vi "WFM MNGR Initialize ET Waveforms.vi"(8 "error in (no error)":errorcluster, 10 "Sequence File":refnum<k7>, 11 "WFM MNGR in":refnum<class "QPA MSMT Waveform Manager.lvclass">) -> (0 "error out":errorcluster, 3 "WFM MNGR out":refnum<class "QPA MSMT Waveform Manager.lvclass">)   [LabVIEW 2016, in "QPA MSMT Waveform Manager.lvclass"]
uses:
  QPA MSMT Waveform Manager.lvclass
  Controls/ET Waveform.ctl
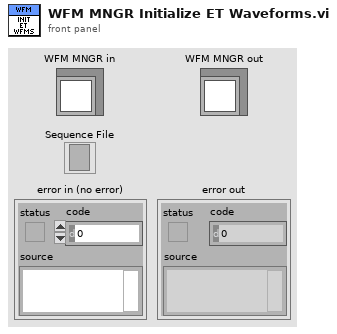
[diagram p1: front panel]
types:
  T1 = typedef "QPA MSMT Waveform Manager.lvclass/ET Waveform.ctl" = cluster{"Name":string, "Path":path, "Vmin":dbl, "Vmax":dbl}
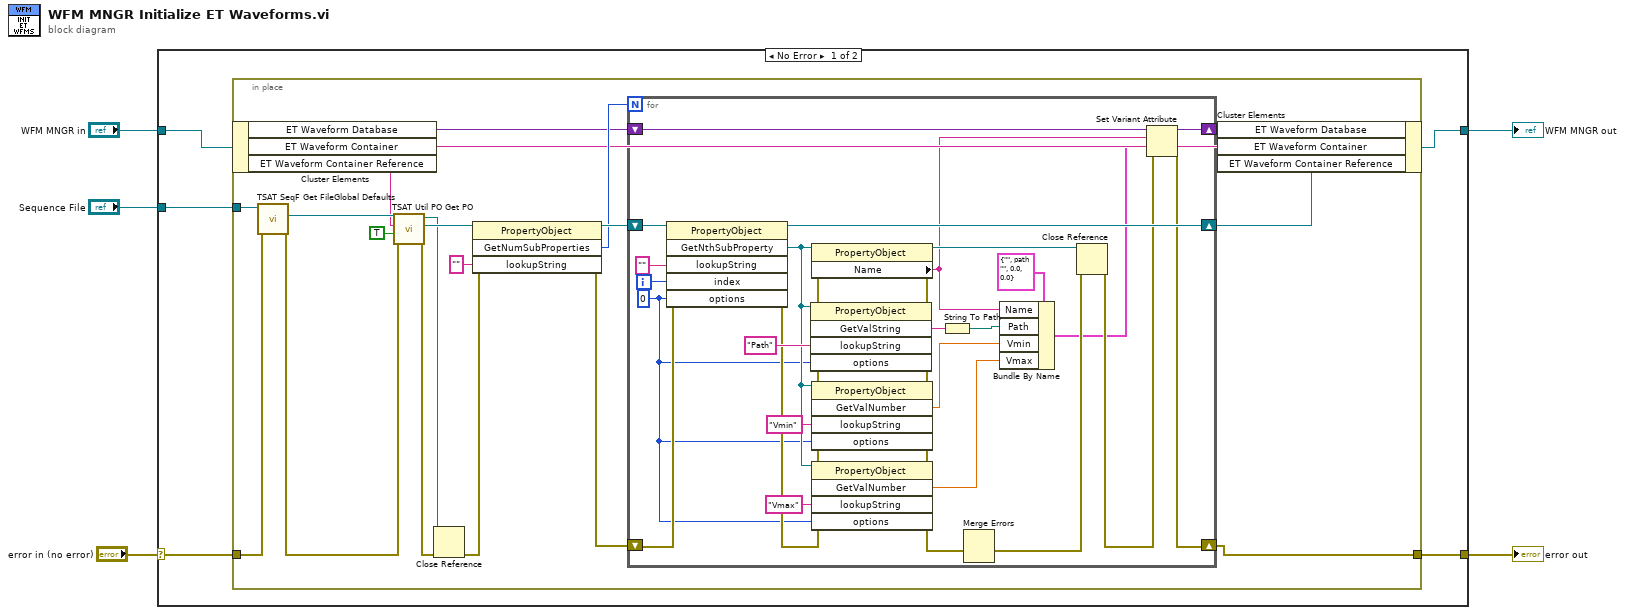
[diagram p0: block diagram]
diagram:
  n1 = case shown="No Error" "error in (no error)" {
    selector: "error in (no error)" -> [w9 w58]
    tunnel: [w6 w58] -> w4
    tunnel: [w7 w57] -> w2
    tunnel: "WFM MNGR in" -> [w8 w57]
    tunnel: "Sequence File" -> [w10 _]
    frame No Error {
      n2 = in-place {
        in-place-border: w10 -> [w19]
        in-place-border: w9 -> [w18]
        in-place-border: [w20] -> w6
        n3 = in-place-cluster #1(w8) -> ("ET Waveform Database"=w17:variant, "ET Waveform Container"=w12:string)  [unwired: 1 out]
        n4 = call "TSAT SeqF Get FileGlobal Defaults.vi"("Error In"=w18, "Sequence File In"=w19) -> ("Error Out"=w27:errorcluster, "FileGlobalsDefaultValues"=w28:refnum<k7>)  [unwired: 7 in, 1 out]
        n5 = call "TSAT Util PO Get PO.vi"("error in (no error)"=w27, "Create if Doesn't Exist?(F)"=TRUE, "Sub Property to Retrieve"=w12, "Property Object in"=w28) -> ("error out"=w25:errorcluster, "SubProperty"=w26:refnum<k7>, "PropertyObjectOut"=w14:refnum<k7>)  [unwired: 5 in]
        n6 = Close Reference(reference=w14, error in (no error)=w25) -> (error out=w15:errorcluster)
        n7 = invoke class="PropertyObject" method="GetNumSubProperties"(reference=w26, error in=w15, "lookupString"="") -> (reference out=w23:refnum<k7>, error out=w21:errorcluster, "GetNumSubProperties"=w22:i32)  [unwired: 1 in, 1 out]
        n8 = for {
          N: w22 -> [_]
          shift-right: [w54] -> w11
          shift-left: w23 -> [w55]
          shift-right: [w32] -> w20
          shift-left: w21 -> [w53]
          shift-right: [w34] -> w16
          shift-left: w17 -> [w35]
          i -> [w56]
          w41 = 0 ("options")
          n9 = invoke class="PropertyObject" method="GetNthSubProperty"(reference=w55, error in=w53, "lookupString"="", "index"=w56, "options"=w41) -> (reference out=w54:refnum<k7>, error out=w44:errorcluster, "GetNthSubProperty"=w45:refnum<k7>)  [unwired: 1 in, 3 out]
          n10 = invoke class="PropertyObject" method="GetValString"(reference=w45, error in=w44, "lookupString"="Path", "options"=w41) -> (error out=w38:errorcluster, "GetValString"=w49:string)  [unwired: 1 in, 3 out]
          n11 = property class="PropertyObject"(reference=w45, error in=w44) -> (reference out=w51:refnum<k7>, error out=w39:errorcluster, "Name"=w30:string)
          n12 = invoke class="PropertyObject" method="GetValNumber"(reference=w45, error in=w44, "lookupString"="Vmin", "options"=w41) -> (error out=w37:errorcluster, "GetValNumber"=w47:dbl)  [unwired: 1 in, 3 out]
          n13 = invoke class="PropertyObject" method="GetValNumber"(reference=w45, error in=w44, "lookupString"="Vmax", "options"=w41) -> (error out=w36:errorcluster, "GetValNumber"=w43:dbl)  [unwired: 1 in, 3 out]
          n14 = String To Path(string=w49) -> (path=w50:path)
          n15 = Merge Errors(w39, w38, w37, w36) -> (w40:errorcluster)
          n16 = Bundle By Name(cluster=T1 {"Name"="", "Path"=path "", "Vmin"=0.0, "Vmax"=0.0} ("RF Waveform"), "Name"=w30, "Path"=w50, "Vmin"=w47, "Vmax"=w43) -> (w31:T1)
          n17 = Close Reference(reference=w51, error in (no error)=w40) -> (error out=w33:errorcluster)
          n18 = Set Variant Attribute(Variant=w35, name=w30, value=w31, error in=w33) -> (Variant out=w34:variant, error out=w32:errorcluster)  [unwired: 1 out]
        }
        n19 = in-place-cluster #1("ET Waveform Database"=w16, "ET Waveform Container"=w12, "ET Waveform Container Reference"=w11) -> (w7:refnum<class "QPA MSMT Waveform Manager.lvclass">)
      }
    }
    frame Error {
    }
  }
  "error out" <- w4
  "WFM MNGR out" <- w2
